vi "TestManager.vi"() -> ()   [LabVIEW 2018]
doc: "This is the central application/framework that controls module, run scripts, etc"
uses:
  TestConfigurationActions.ctl
  LV_Config_class/Config.lvclass/Config.ctl
  VisualizationManagement/VisualizationManagerActions.ctl
  NistPluggableModules/TestClass/Test.lvclass/Test.ctl
  <vilib>/Utility/miscctls.llb/LVRowAndColumnTypeDef.ctl
  LV_Config_class/Accessors/Read ConfigFilePath.vi
  LV_Config_class/Accessors/Write ConfigFilePath.vi
  NistPluggableModules/TestClass/Accessors/Read ModuleList.vi
  <vilib>/Utility/error.llb/Error Cluster From Error Code.vi
  <vilib>/ErrorRing/Error Ring.xnode
  Queue/Queue.lvlib
  <userlib>/NIST/NISTErrorLib/NISTErrorLib.lvlib
  LV_Config_class/Config.lvclass
  <vilib>/Utility/config.llb/NI_LVConfig.lvlib
  Message Queue/Message Queue.lvlib
  NistPluggableModules/TestClass/Test.lvclass
  LV_TestAutomation/Comms_lib/Comms.lvlib
panel:
  in  "Error In":errorcluster
  in  "Create Error (Test Python Multirun)":bool
  out "Test Tree Caption":string="Test Configuration"
  in  "btnClearTest":bool
  in  "btnSaveTestTree":bool
  in  "btnSaveTestAs":bool
  in  "btnLoadTest":bool
  in  "btnStopAllRunningTests":bool
  in  "btnRunAll":bool
  in  "TestTree":i32[](listbox)
  out "tstFilePath":path
  in  "Stop?":bool
  in  "btnRunScript":bool
  in  "btnDelete":bool
  out "OrigTestTreeTags":string[](array[string])
  out "Test Script":string
  in  "Experiment Specific Controls":T1(tab)
  in  "Priority":u8=2
  in  "Severity":string="Abort"
  out "Error Out":errorcluster
  in  "Severity":string
  in  "Priority":u8=2
  in  "Create Error (Test AutoTimeout)":bool
  in  "Error In 2":errorcluster
  # "Test Script Preview"
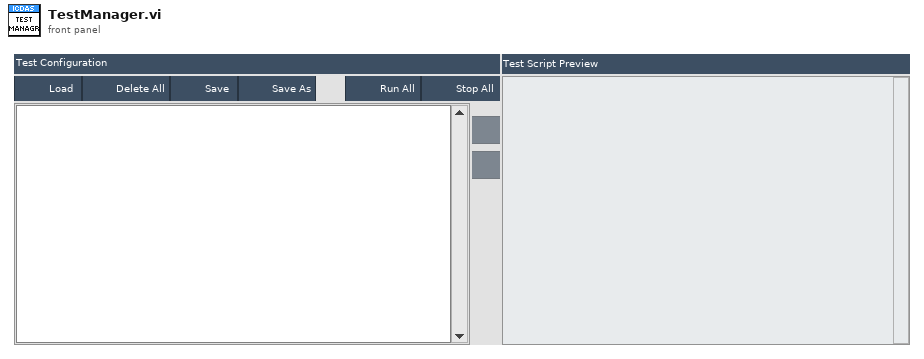
[diagram p1: front panel]
types:
  T1 = enum32{"PV Aging Experiment", "Pacific Power ", "Miscellaneous ", "Errors", "Test AutoTimeout", "Test Python MutliRun"}
  T2 = typedef "clUserEvents.ctl" = cluster{"StopEvent":refnum<user-event>, "RefreshUserEvents":refnum<user-event>, "StatusUpdate":refnum<user-event>, "RunAllScripts":refnum<user-event>}
  T3 = typedef "Message Queue.lvlib/All Message Queues.ctl" = cluster{"UI":refnum<queue>}
  T4 = typedef "cntlRefs.ctl" = cluster{"rngFGen":refnum<vi>, "rngDigitizer":refnum<vi>, "btnHide":refnum<vi>, "rngInst":refnum<vi>, "Instrument Modules":refnum<vi>, "RelativePathToINIFiles ":refnum<vi>, "PluginTree":refnum<vi>, "TestListboxRef":refnum<vi>, "path.tstFile":refnum<vi>, "cmbxRunningModules":refnum<vi>, "TestDataSubPanel":refnum<vi>, "TestDataCaption":refnum<vi>, "btnPopInOut":refnum<vi>, "PluginMgrQ":refnum<queue>, "TestMgrQ":refnum<queue>, "TestMgrSubPanel":refnum<vi>, "PluginMgrSubPanel":refnum<vi>, "PwrReqHandle":u32, "btnStopOneTest":refnum<vi>, "pathUserfiles":refnum<vi>, "PluginTreeCaption":refnum<vi>}
  T5 = enum8{"Enabled", "Disabled", "Disabled and Grayed Out"}
  T6 = typedef "TestConfigurationActions.ctl" = enum16{"Save", "Save As", "Read", "Read&Load"}
  T7 = typedef "VisualizationManagerActions.ctl" = enum16{"Set", "LoadModVI", "PopInOutModVI", "Add", "Clear", "CloseVisMod"}
  T8 = typedef "LVRowAndColumnTypeDef.ctl" = cluster{"Row":i32, "Column":i32}
  T9 = typedef "NI_LVConfig.lvlib/Config Data RefNum.ctl" = refnum<k1>
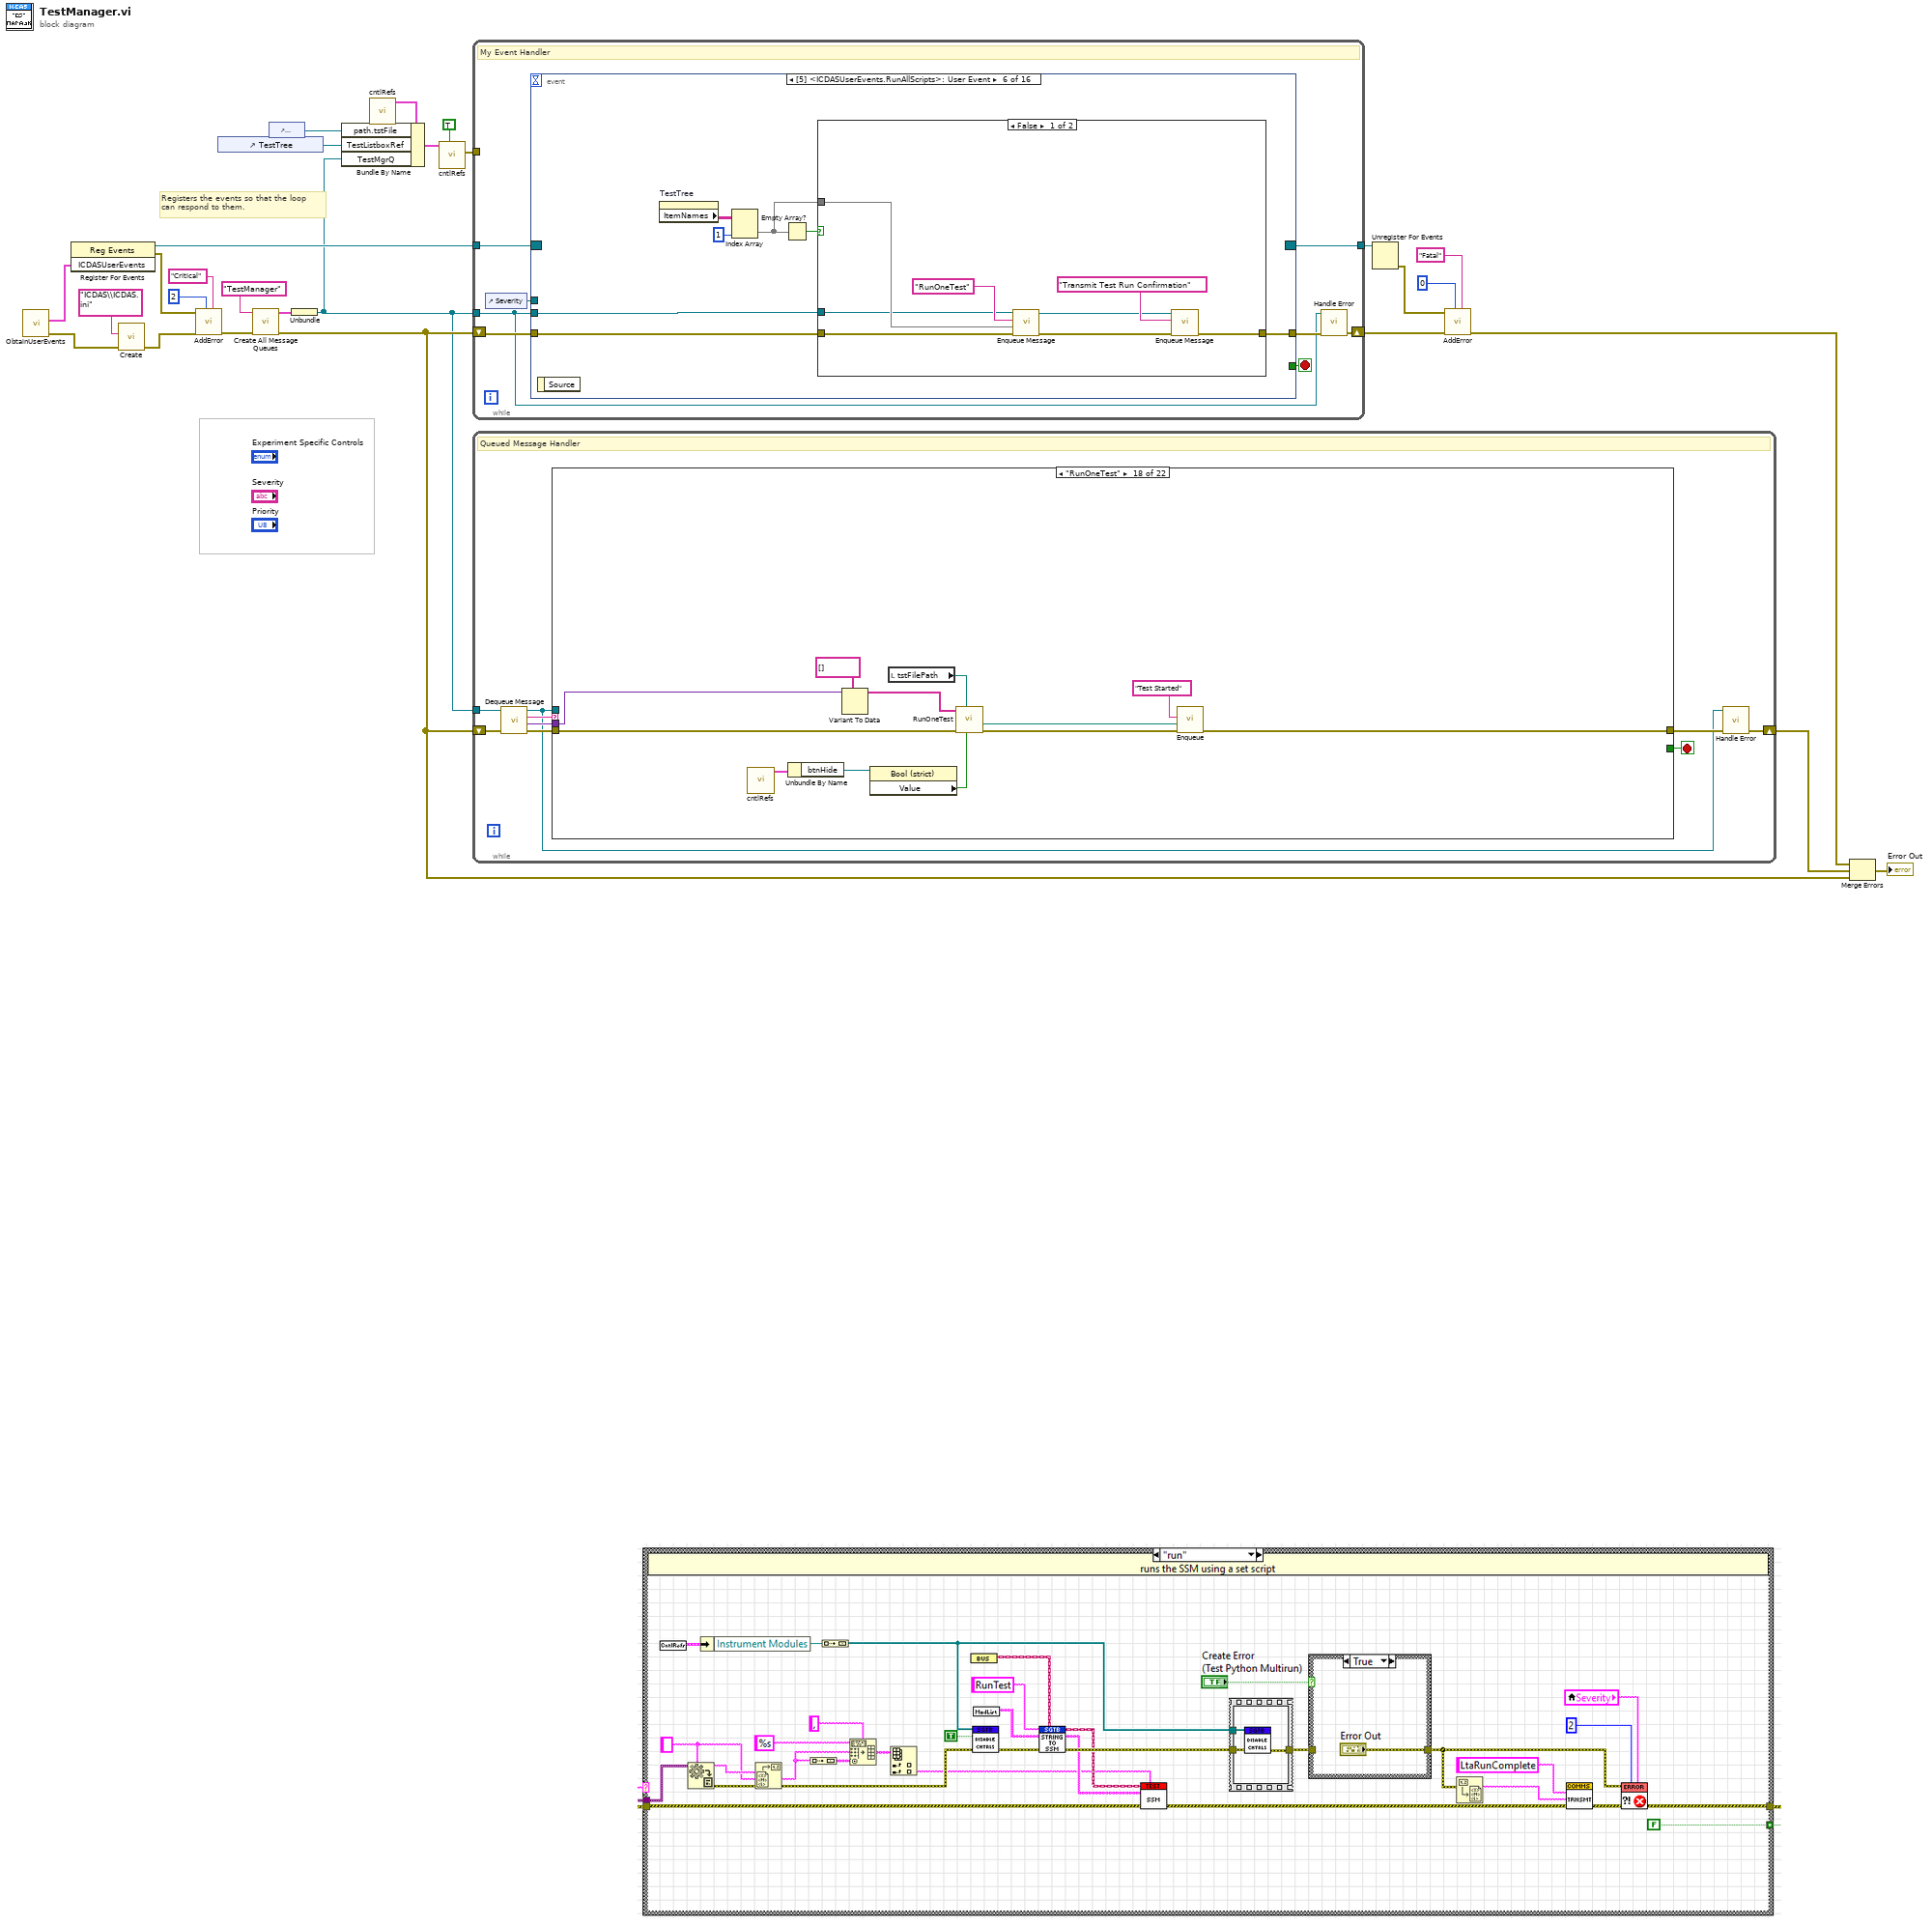
[diagram p0: block diagram]
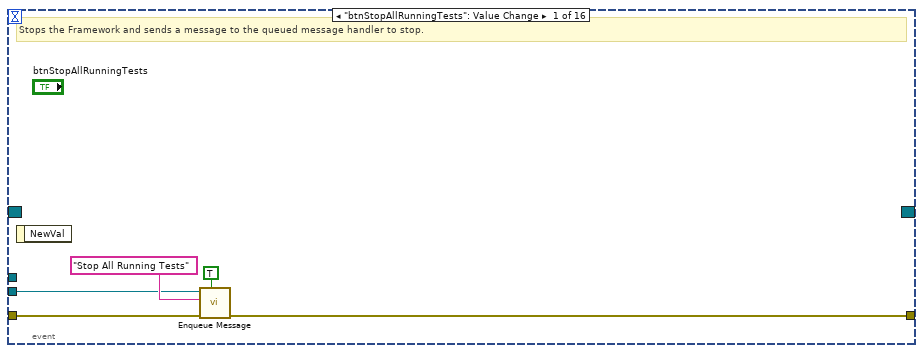
[diagram p2: hidden frame]
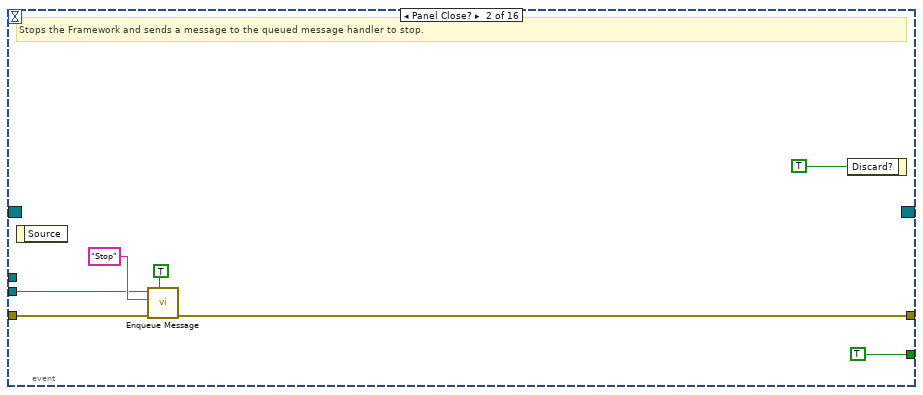
[diagram p3: hidden frame]
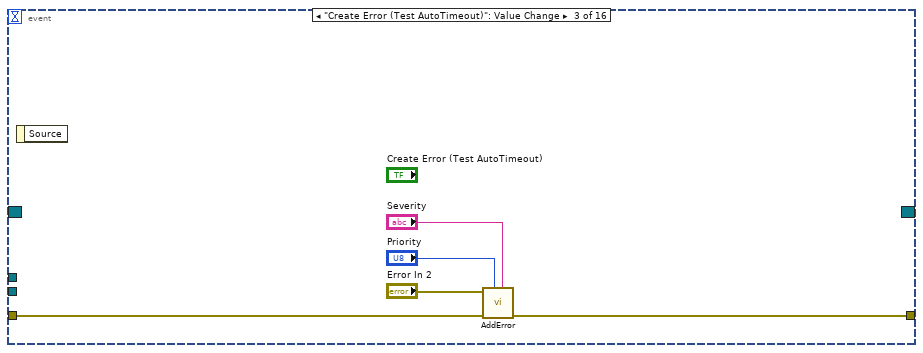
[diagram p4: hidden frame]
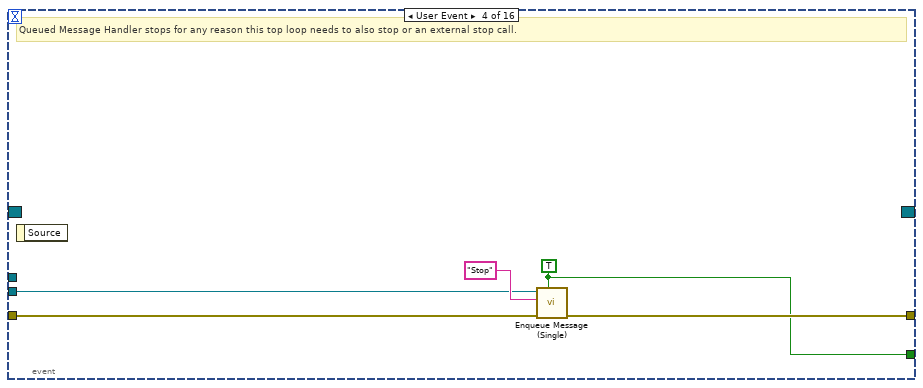
[diagram p5: hidden frame]
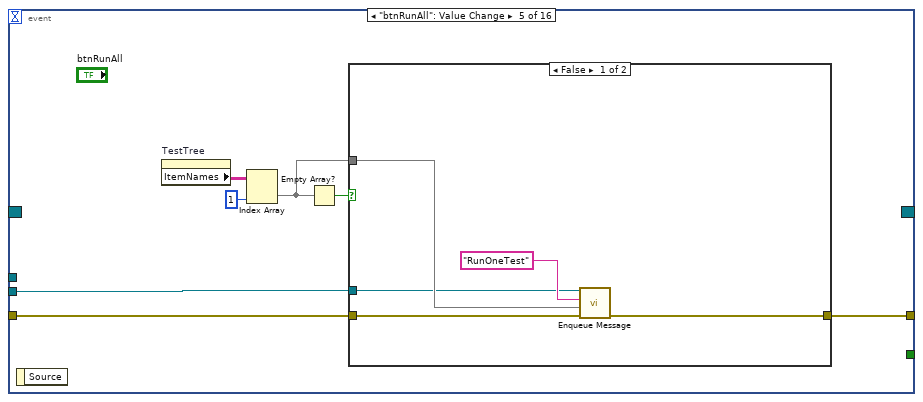
[diagram p6: hidden frame]
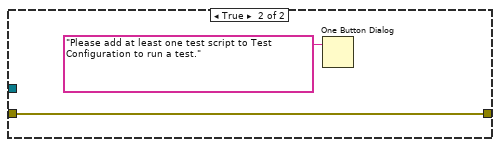
[diagram p7: hidden frame]
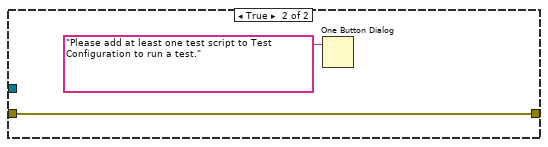
[diagram p8: hidden frame]
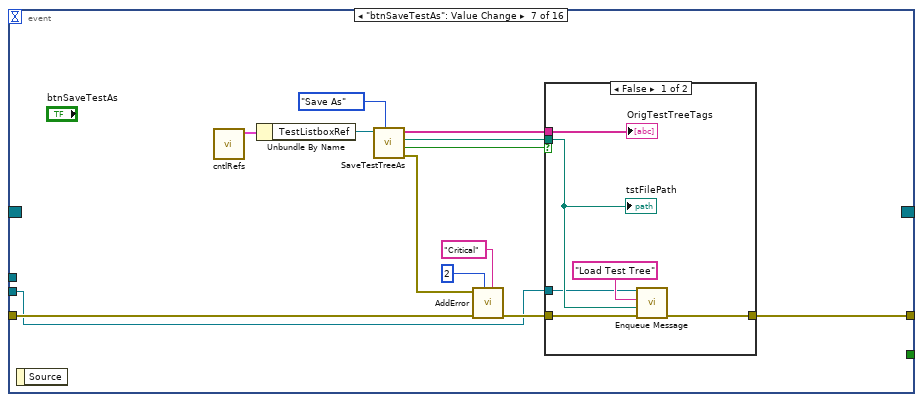
[diagram p9: hidden frame]
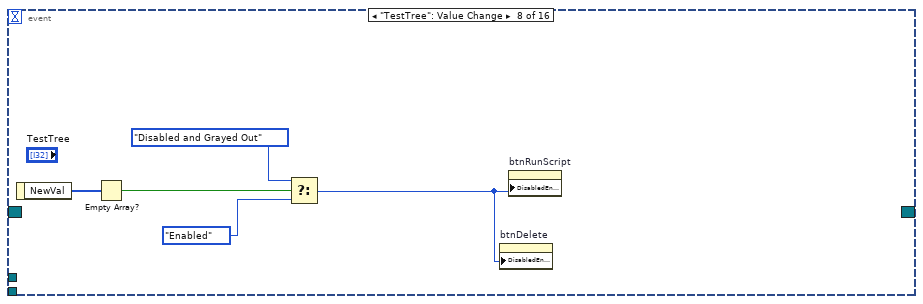
[diagram p11: hidden frame]
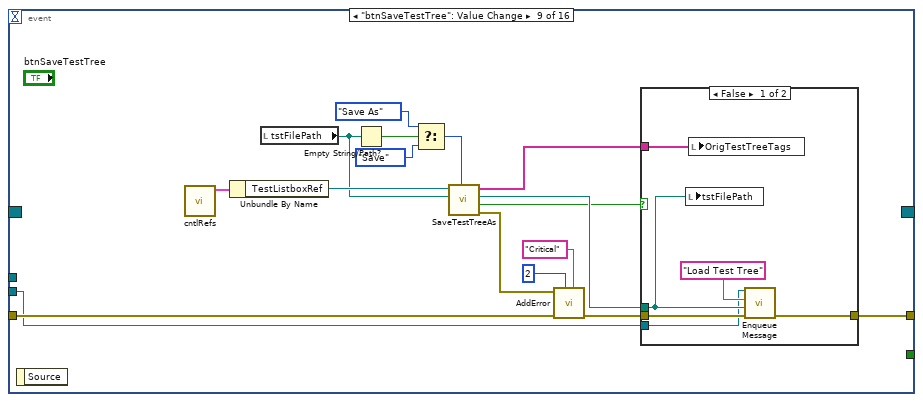
[diagram p12: hidden frame]
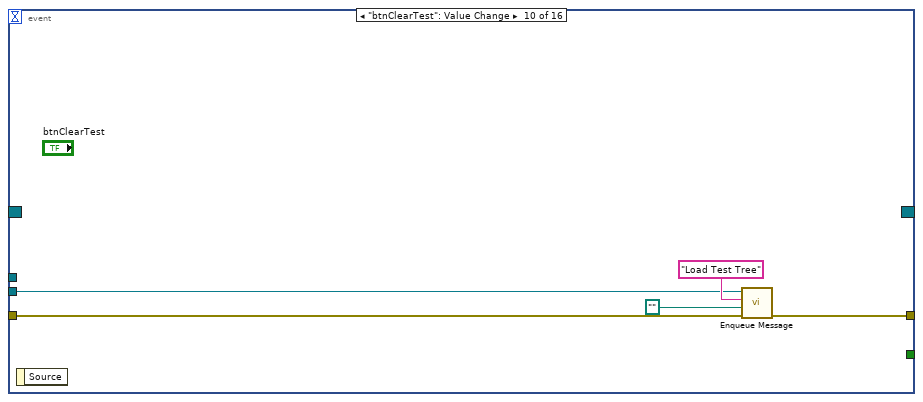
[diagram p14: hidden frame]
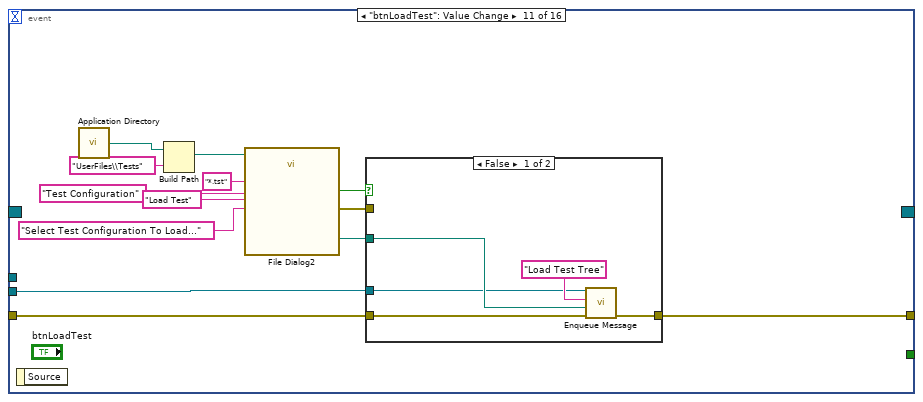
[diagram p15: hidden frame]
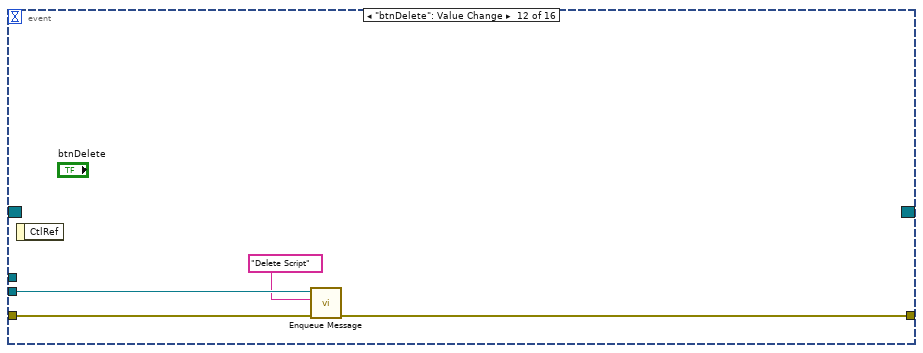
[diagram p17: hidden frame]
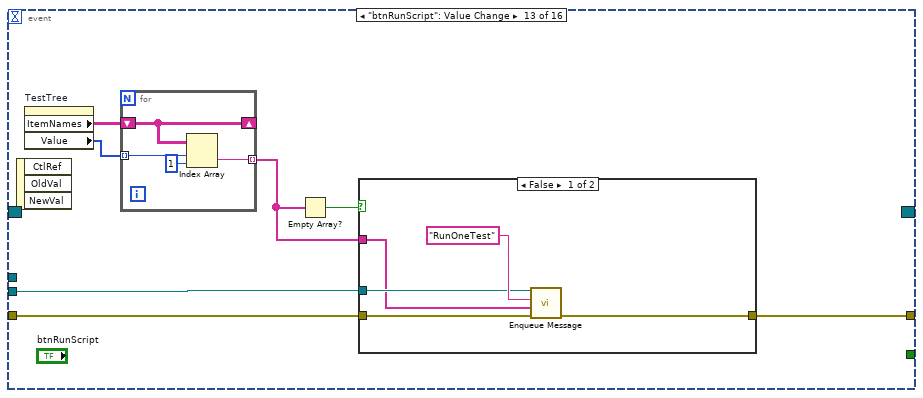
[diagram p18: hidden frame]
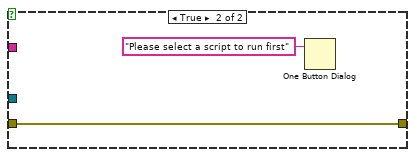
[diagram p19: hidden frame]
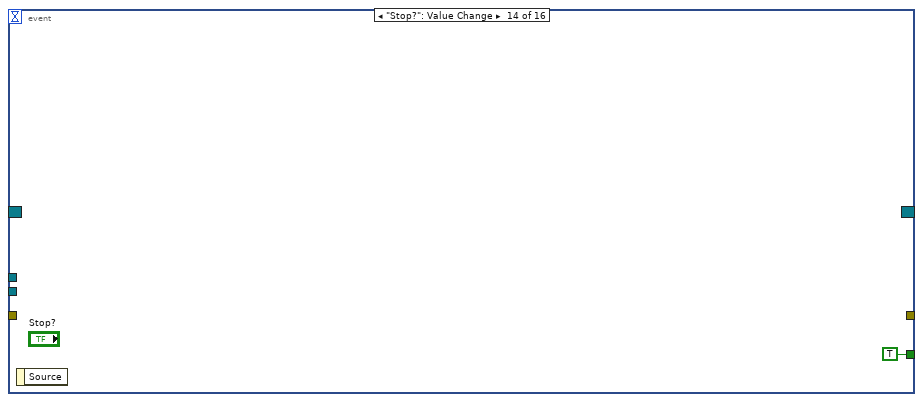
[diagram p20: hidden frame]
diagram:
  # "Registers the events so that the loop \ncan respond to them."
  n1 = call "ObtainUserEvents.vi"() -> ("ErrorArray"=w8:errorcluster[], "ICDASUserEvents"=w26:T2)  [unwired: 10 in]
  n2 = register-events(w26) -> (reference out=w27:refnum<event-registration>, error out=w16:errorcluster)  [unwired: 2 in]
  n3 = call "Create.vi"("ErrorArray"=w8, "name or relative path"="ICDAS\\ICDAS.ini") -> ("ErrorArray"=w7:errorcluster[])  [unwired: 8 in, 1 out]
  n4 = call <userlib>:"AddError.vi"("Severity"="Critical", "Priority"=u8 2, "ErrorArray In"=w7, "error in (no error)"=w16) -> ("ErrorArray Out"=w11:errorcluster[])  [unwired: 6 in, 1 out]
  n5 = control-ref of="TestTree"() -> (w15:refnum<vi>)
  n6 = call "Create All Message Queues.vi"("error in (no error)"=w11, "Queue Name (unnamed)"="TestManager") -> ("error out"=w10:errorcluster[], "Message Queues out"=w12:T3)  [unwired: 8 in]
  n7 = control-ref of="tstFilePath"() -> (w14:refnum<vi>)
  n8 = Unbundle(w12) -> ("UI"=w3:refnum<queue>)
  n9 = call "cntlRefs.vi"() -> ("cntlRefs"=w6:T4)  [unwired: 10 in, 1 out]
  n10 = Bundle By Name(cluster=w6, "path.tstFile"=w14, "TestListboxRef"=w15, "TestMgrQ"=w3) -> (w22:T4)
  n11 = call "cntlRefs.vi"("Set?"=TRUE, "cntlRefs"=w22) -> ("error out"=w4:errorcluster[])  [unwired: 8 in, 1 out]
  n12 = while {
    tunnel: w27 -> [w35]
    shift-right: [w33] -> w18
    shift-left: w10 -> [w34]
    tunnel: w3 -> [w29]
    tunnel: w4 -> [_]
    tunnel: [w28] -> w2
    stop <- w32 stop-if-true
    # "My Event Handler"
    n13 = control-ref of="Severity"() -> (w31:refnum<vi>)
    n14 = event shown="[5] <ICDASUserEvents.RunAllScripts>: User Event" {
      selector: w35 -> [_ _ _ _ _ _ _ _ _ _ _ _ _ _ _ _]
      dyn-events: [_ _ _ _ _ _ _ _ _ _ _ _ _ _ _ _] -> w28
      timeout: _ -> [_ _ _ _ _ _ _ _ _ _ _ _ _ _ _ _]
      tunnel: w34 -> [w40 w47 w51 w56 w63 w77 w96 _ w126 w142 w155 w164 w172 _ w188 w205]
      tunnel: [w37 w46 w50 w55 w62 w76 w93 _ w117 w141 w154 w165 w171 _ w187 w203] -> w30
      tunnel: [_ TRUE ("Priority (F)") _ w54 _ _ _ _ _ _ _ _ _ TRUE ("Priority (F)") _ _] -> w32
      tunnel: w31 -> [_ _ _ _ _ _ _ _ _ _ _ _ _ _ _ _]
      tunnel: w29 -> [w36 w41 _ w53 w61 w75 w89 _ w114 w138 w143 w163 w170 _ w186 w204]
      event "btnStopAllRunningTests": Value Change {
        # "Stops the Framework and sends a message to the queued message handler to stop."
        n15 = event-data() -> ()  [unwired: 1 in, 1 out]
        n16 = call-poly "Enqueue Message.vi"("Priority Message? (F)"=TRUE ("Priority (F)"), "error in (no error)"=w40, "Message"="Stop All Running Tests", "Message Queue"=w36) -> ("error out"=w37:errorcluster[])  [unwired: 6 in, 1 out]
      }
      event Panel Close? {
        # "Stops the Framework and sends a message to the queued message handler to stop."
        n17 = event-data() -> ()  [unwired: 1 in, 1 out]
        n18 = call-poly "Enqueue Message.vi"("Priority Message? (F)"=TRUE ("Priority (F)"), "error in (no error)"=w47, "Message"="Stop", "Message Queue"=w41) -> ("error out"=w46:errorcluster[])  [unwired: 6 in, 1 out]
        n19 = event-data("Discard?"=TRUE) -> ()  [unwired: 1 in, 1 out]
      }
      event "Create Error (Test AutoTimeout)": Value Change {
        n20 = event-data() -> ()  [unwired: 1 in, 1 out]
        n21 = call <userlib>:"AddError.vi"("Severity"="Severity", "Priority"="Priority", "ErrorArray In"=w51, "error in (no error)"="Error In 2") -> ("ErrorArray Out"=w50:errorcluster[])  [unwired: 6 in, 1 out]
      }
      event User Event {
        w54 = TRUE ("Priority (F)")
        # "Queued Message Handler stops for any reason this top loop needs to also stop or an external stop call."
        n22 = event-data() -> ()  [unwired: 1 in, 1 out]
        n23 = call "Enqueue Message (Single).vi"("Priority Message? (F)"=w54, "error in (no error)"=w56, "Message"="Stop", "Message Queue"=w53) -> ("error out"=w55:errorcluster[])  [unwired: 6 in, 1 out]
      }
      event "btnRunAll": Value Change {
        n24 = event-data() -> ()  [unwired: 1 in, 1 out]
        n25 = property on="TestTree" class="MCListbox (strict)"() -> ("ItemNames"=w60:string[][])  [unwired: 2 in, 2 out]
        n26 = Index Array(array=w60, index (col)=1 ("disabled index (col)")) -> (element=w58:string[])  [unwired: 1 in]
        n27 = Empty Array?(array=w58) -> (empty?=w64:bool)
        n28 = case shown="False" w64 {
          tunnel: w58 -> [w67 _]
          tunnel: w63 -> [w69 w70]
          tunnel: [w65 w70] -> w62
          tunnel: w61 -> [w66 _]
          frame False {
            n29 = call-poly "Enqueue Message.vi"("error in (no error)"=w69, "Message Data"=w67, "Message"="RunOneTest", "Message Queue"=w66) -> ("error out"=w65:errorcluster[])  [unwired: 6 in, 1 out]
          }
          frame True {
            n30 = One Button Dialog(message="Please add at least one test script to Test Configuration to run a test.") -> ()  [unwired: 1 in, 1 out]
          }
        }
      }
      event User Event {
        n31 = event-data() -> ()  [unwired: 1 in, 1 out]
        n32 = property on="TestTree" class="MCListbox (strict)"() -> ("ItemNames"=w74:string[][])  [unwired: 2 in, 2 out]
        n33 = Index Array(array=w74, index (col)=1 ("disabled index (col)")) -> (element=w72:string[])  [unwired: 1 in]
        n34 = Empty Array?(array=w72) -> (empty?=w78:bool)
        n35 = case shown="False" w78 {
          tunnel: w72 -> [w84 _]
          tunnel: w77 -> [w86 w87]
          tunnel: [w79 w87] -> w76
          tunnel: w75 -> [w83 _]
          frame False {
            n36 = call-poly "Enqueue Message.vi"("error in (no error)"=w86, "Message Data"=w84, "Message"="RunOneTest", "Message Queue"=w83) -> ("error out"=w80:errorcluster[], "dup Message Queue"=w81:refnum<queue>)  [unwired: 6 in]
            n37 = call-poly "Enqueue Message.vi"("error in (no error)"=w80, "Message"="Transmit Test Run Confirmation", "Message Queue"=w81) -> ("error out"=w79:errorcluster[])  [unwired: 7 in, 1 out]
          }
          frame True {
            n38 = One Button Dialog(message="Please add at least one test script to Test Configuration to run a test.") -> ()  [unwired: 1 in, 1 out]
          }
        }
      }
      event "btnSaveTestAs": Value Change {
        n39 = event-data() -> ()  [unwired: 1 in, 1 out]
        n40 = call "cntlRefs.vi"() -> ("cntlRefs"=w101:T4)  [unwired: 10 in, 1 out]
        n41 = Unbundle By Name(w101) -> ("TestListboxRef"=w100:refnum<vi>)
        n42 = call "SaveTestTreeAs.vi"("Action"=enum16{"Save", "Save As"}."Save As", "ListboxRef"=w100) -> ("error out"=w95:errorcluster, "Cancelled?"=w90:bool, "path.tstFile"=w92:path, "All Test Tree Tags"=w91:string[])  [unwired: 5 in, 1 out]
        n43 = call <userlib>:"AddError.vi"("Severity"="Critical", "Priority"=u8 2, "ErrorArray In"=w96, "error in (no error)"=w95) -> ("ErrorArray Out"=w94:errorcluster[])  [unwired: 6 in, 1 out]
        n44 = case shown="False" w90 {
          tunnel: w94 -> [w106 w108]
          tunnel: [w105 w108] -> w93
          tunnel: w92 -> [w104 _]
          tunnel: w91 -> [w103 _]
          tunnel: w89 -> [w102 _]
          frame False {
            n45 = call-poly "Enqueue Message.vi"("error in (no error)"=w106, "Message Data"=w104, "Message"="Load Test Tree", "Message Queue"=w102) -> ("error out"=w105:errorcluster[])  [unwired: 6 in, 1 out]
            "tstFilePath" <- w104
            "OrigTestTreeTags" <- w103
          }
          frame True {
          }
        }
      }
      event "TestTree": Value Change {
        n46 = event-data() -> ("NewVal"=w113:i32[])  [unwired: 1 in]
        n47 = Empty Array?(array=w113) -> (empty?=w112:bool)
        n48 = Select(t=T5."Disabled and Grayed Out" ("Disabled"), s=w112, f=T5."Enabled" ("Disabled")) -> (s? t:f=w109:T5)
        n49 = property on="btnDelete" class="Bool"("DisabledEnum"=w109) -> ()  [unwired: 2 in, 2 out]
        n50 = property on="btnRunScript" class="Bool"("DisabledEnum"=w109) -> ()  [unwired: 2 in, 2 out]
      }
      event "btnSaveTestTree": Value Change {
        n51 = event-data() -> ()  [unwired: 1 in, 1 out]
        n52 = call "cntlRefs.vi"() -> ("cntlRefs"=w129:T4)  [unwired: 10 in, 1 out]
        n53 = Unbundle By Name(w129) -> ("TestListboxRef"=w130:refnum<vi>)
        n54 = local read "tstFilePath"() -> (w124:path)
        n55 = Empty String/Path?(string/path=w124) -> (empty?=w123:bool)
        n56 = Select(t=TestConfigurationActions."Save As" ("Action"), s=w123, f=TestConfigurationActions."Save" ("Action")) -> (s? t:f=w120:T6)
        n57 = call "SaveTestTreeAs.vi"("Action"=w120, ".tst File Path"=w124, "ListboxRef"=w130) -> ("error out"=w125:errorcluster, "Cancelled?"=w115:bool, "path.tstFile"=w116:path, "All Test Tree Tags"=w119:string[])  [unwired: 4 in, 1 out]
        n58 = call <userlib>:"AddError.vi"("Severity"="Critical", "Priority"=u8 2, "ErrorArray In"=w126, "error in (no error)"=w125) -> ("ErrorArray Out"=w118:errorcluster[])  [unwired: 6 in, 1 out]
        n59 = case shown="False" w115 {
          tunnel: w119 -> [w136 _]
          tunnel: w118 -> [w134 w137]
          tunnel: [w133 w137] -> w117
          tunnel: w116 -> [w132 _]
          tunnel: w114 -> [w131 _]
          frame False {
            n60 = local write "tstFilePath"(w132) -> ()
            n61 = local write "OrigTestTreeTags"(w136) -> ()
            n62 = call-poly "Enqueue Message.vi"("error in (no error)"=w134, "Message Data"=w132, "Message"="Load Test Tree", "Message Queue"=w131) -> ("error out"=w133:errorcluster[])  [unwired: 6 in, 1 out]
          }
          frame True {
          }
        }
      }
      event "btnClearTest": Value Change {
        n63 = event-data() -> ()  [unwired: 1 in, 1 out]
        n64 = call-poly "Enqueue Message.vi"("error in (no error)"=w142, "Message Data"=path "", "Message"="Load Test Tree", "Message Queue"=w138) -> ("error out"=w141:errorcluster[])  [unwired: 6 in, 1 out]
      }
      event "btnLoadTest": Value Change {
        n65 = event-data() -> ()  [unwired: 1 in, 1 out]
        n66 = call <vilib>:"Application Directory.vi"() -> ("Application Directory"=w152:path)
        n67 = Build Path(base path=w152, name or relative path="UserFiles\\Tests") -> (appended path=w150:path)
        n68 = call "File Dialog2"("start path"=w150, "prompt"="Select Test Configuration To Load...", "button label"="Load Test", "pattern (all files)"="*.tst", "pattern label"="Test Configuration") -> ("selected path"=w145:path, "cancelled"=w144:bool, "error out"=w146:errorcluster)  [unwired: 7 in, 1 out]
        n69 = case shown="False" w144 {
          tunnel: w155 -> [w160 w161]
          tunnel: [w158 w161] -> w154
          tunnel: w146 -> [_ _]
          tunnel: w145 -> [w157 _]
          tunnel: w143 -> [w156 _]
          frame False {
            n70 = call-poly "Enqueue Message.vi"("error in (no error)"=w160, "Message Data"=w157, "Message"="Load Test Tree", "Message Queue"=w156) -> ("error out"=w158:errorcluster[])  [unwired: 6 in, 1 out]
          }
          frame True {
          }
        }
      }
      event "btnDelete": Value Change {
        n71 = event-data() -> ()  [unwired: 1 in, 1 out]
        n72 = call-poly "Enqueue Message.vi"("error in (no error)"=w164, "Message"="Delete Script", "Message Queue"=w163) -> ("error out"=w165:errorcluster[])  [unwired: 7 in, 1 out]
      }
      event "btnRunScript": Value Change {
        n73 = event-data() -> ()  [unwired: 1 in, 3 out]
        n74 = property on="TestTree" class="MCListbox (strict)"() -> ("ItemNames"=w169:string[][], "Value"=w168:i32[])  [unwired: 2 in, 2 out]
        n75 = for {
          shift-right: [w175] -> _
          shift-left: w169 -> [w175]
          tunnel: w168 -> [w176] mode=indexing
          tunnel: [w173] -> w167 mode=indexing
          n76 = Index Array(array=w175, index (row)=w176, index (col)=1 ("disabled index (col)")) -> (element=w173:string)
        }
        n77 = Empty Array?(array=w167) -> (empty?=w166:bool)
        n78 = case shown="False" w166 {
          tunnel: w172 -> [w181 w183]
          tunnel: [w180 w183] -> w171
          tunnel: w170 -> [w178 _]
          tunnel: w167 -> [w177 _]
          frame False {
            n79 = call-poly "Enqueue Message.vi"("error in (no error)"=w181, "Message Data"=w177, "Message"="RunOneTest", "Message Queue"=w178) -> ("error out"=w180:errorcluster[])  [unwired: 6 in, 1 out]
          }
          frame True {
            n80 = One Button Dialog(message="Please select a script to run first") -> ()  [unwired: 1 in, 1 out]
          }
        }
      }
      event "Stop?": Value Change {
        n81 = event-data() -> ()  [unwired: 1 in, 1 out]
      }
      event "TestTree": Drag Ended {
        n82 = event-data() -> ("Result"=w185:enum16{"Drop Cancel", "Drop Move", "Drop Copy"})  [unwired: 1 in]
        n83 = case shown="\"Drop Move\"" w185 {
          tunnel: w188 -> [w189 w195]
          tunnel: [w189 w194] -> w187
          tunnel: w186 -> [_ w193]
          frame "Drop Cancel", Default {
          }
          frame "Drop Move" {
            # "Refresh Test Script Preview"
            n84 = property on="TestTree" class="MCListbox (strict)"() -> ("ItemNames"=w192:string[][])  [unwired: 2 in, 2 out]
            n85 = Index Array(array=w192, index (col)=1 ("disabled index (col)")) -> (element=w190:string[])  [unwired: 1 in]
            n86 = local read "OrigTestTreeTags"() -> (w201:string[])
            n87 = call "CheckIfStringArraysAreEqual-1D.vi"("Array2"=w190, "Array1"=w201) -> ("Equal?"=w200:bool)  [unwired: 9 in]
            n88 = Not(x=w200) -> (.not. x?=w199:bool)
            n89 = call-poly "Enqueue Message.vi"("error in (no error)"=w195, "Message Data"=w199, "Message"="Test Tree Save State", "Message Queue"=w193) -> ("error out"=w202:errorcluster[], "dup Message Queue"=w198:refnum<queue>)  [unwired: 6 in]
            n90 = call-poly "Enqueue Message.vi"("error in (no error)"=w202, "Message"="Refresh Test Script", "Message Queue"=w198) -> ("error out"=w194:errorcluster[])  [unwired: 7 in, 1 out]
          }
        }
      }
      event Pane Size {
        n91 = event-data() -> ()  [unwired: 1 in, 6 out]
        n92 = call "Enqueue Message (Single).vi"("error in (no error)"=w205, "Message"="Resize Test Listbox Column", "Message Queue"=w204) -> ("error out"=w203:errorcluster[])  [unwired: 7 in, 1 out]
      }
    }
    n93 = call "Handle Error.vi"("ErrorArrayIn"=w30, "Message Queue"=w29) -> ("ErrorArrayOut"=w33:errorcluster[])  [unwired: 9 in]
  }
  n94 = while {
    shift-right: [w214] -> w21
    shift-left: w10 -> [w209]
    tunnel: w3 -> [w212]
    stop <- w213 stop-if-true
    # "Queued Message Handler"
    n95 = call "Dequeue Message.vi"("error in (no error)"=w209, "Message Queue"=w212) -> ("error out"=w208:errorcluster[], "Message Data"=w211:variant, "Message"=w210:string, "dup Message Queue"=w207:refnum<queue>)  [unwired: 6 in]
    n96 = case shown="\"RunOneTest\"" w210 {
      selector: w210 -> [_ _ _ _ _ _ w377 _ _ _ _ _ _ _ _ _ _ _ _ _ _ _]
      tunnel: [w229 w266 w269 w311 w356 w368 w376 w385 w394 w398 w411 w472 w476 w481 w503 w505 w548 w550 w562 w569 w576 w583] -> w215
      tunnel: w208 -> [w236 w265 w274 w310 w351 w359 w375 w385 w394 w397 w431 w471 w476 w482 w503 w515 w548 w556 w564 w568 w576 w583]
      tunnel: [_ _ _ _ _ TRUE _ _ _ _ _ _ _ _ _ _ _ _ _ _ _ _] -> w213
      tunnel: w211 -> [_ w264 w275 _ w355 _ _ _ w392 _ w425 _ _ w478 _ w514 _ w557 _ _ _ _]
      tunnel: w207 -> [w225 w263 w267 w301 w333 w364 _ _ _ _ w407 w470 _ w480 _ _ _ _ _ _ _ _]
      frame "Initialize" {
        # "Pulls the default configuration from the INI file"
        n97 = call "GetSetConfigClass.vi"() -> ("Ref out"=w234:refnum<class "Config.lvclass">)  [unwired: 11 in]
        n98 = property class="Config.lvclass"(reference=w234) -> ("Accessors:ConfigFilePath"=w231:path)  [unwired: 1 in, 2 out]
        n99 = To Variant(anything=w231) -> (Variant=w230:variant)
        n100 = call "cntlRefs.vi"() -> ("cntlRefs"=w228:T4)  [unwired: 10 in, 1 out]
        n101 = Unbundle By Name(w228) -> ("TestListboxRef"=w224:refnum<vi>)
        n102 = call "Enqueue Message (Single).vi"("error in (no error)"=w236, "Message Data"=w230, "Message"="LoadTest", "Message Queue"=w225) -> ("error out"=w219:errorcluster[], "dup Message Queue"=w217:refnum<queue>)  [unwired: 6 in]
        n103 = call "Enqueue Message (Single).vi"("error in (no error)"=w219, "Message"="Resize Test Listbox Column", "Message Queue"=w217) -> ("error out"=w218:errorcluster[])  [unwired: 7 in, 1 out]
        n104 = property class="MCListbox"(reference=w224, "ItemNames"=string[][] [] ("Item Names")) -> (reference out=w223:refnum<vi>, error out=w221:errorcluster)  [unwired: 1 in]
        n105 = call "ListboxSymbols-FG.vi"("Actions"=enum16{"Init Symbols", "Set Item Symbol"}."Init Symbols", "error in (no error)"=w221, "ListboxRef"=w223) -> ("error out"=w220:errorcluster)  [unwired: 5 in, 3 out]
        n106 = call <userlib>:"AddError.vi"("Severity"="Fatal", "Priority"=u8 0, "ErrorArray In"=w218, "error in (no error)"=w220) -> ("ErrorArray Out"=w229:errorcluster[])  [unwired: 6 in, 1 out]
        "Test Script" <- ""
      }
      frame "LoadTest" {
        # "From the default file load the last saved results and updated the controls and indicators"
        n107 = call "cntlRefs.vi"() -> ("cntlRefs"=w258:T4)  [unwired: 10 in, 1 out]
        n108 = Variant To Data(type=path "", Variant=w264) -> (data=w260:path, error out=w262:errorcluster)  [unwired: 1 in]
        n109 = Unbundle By Name(w258) -> ("path.tstFile"=w257:refnum<vi>)
        n110 = call <vilib>:"Open Config Data.vi"("error in (no error)"=w262, "configuration file path"=w260) -> ("error out"=w241:errorcluster, "refnum"=w259:T9)  [unwired: 7 in, 1 out]
        n111 = property class="Path"(reference=w257, error in=w241) -> (error out=w254:errorcluster, "Label.Text"=w255:string)  [unwired: 1 out]
        n112 = call <userlib>:"Read Key (Variant)__ogtk.vi"("section"=w255, "error in (no error)"=w254, "type"=w255, "key (optional)"=w255, "refnum"=w259) -> ("error out"=w253:errorcluster, "key-value"=w256:variant, "refnum out"=w240:T9)  [unwired: 3 in, 1 out]
        n113 = Variant To Data(error in=w253, type=w255, Variant=w256) -> (data=w252:string, error out=w239:errorcluster)
        n114 = call <vilib>:"Trim Whitespace.vi"("string"=w252) -> ("trimmed string"=w246:string)  [unwired: 1 in]
        n115 = call <vilib>:"Close Config Data.vi"("error in (no error)"=w239, "write file if changed (T)"=FALSE, "refnum"=w240) -> ("error out"=w238:errorcluster)  [unwired: 7 in, 1 out]
        n116 = Empty String/Path?(string/path=w246) -> (empty?=w245:bool)
        n117 = call <vilib>:"Application Directory.vi"() -> ("Application Directory"=w247:path)
        n118 = local read "Severity"() -> (w250:string)
        n119 = local read "Priority"() -> (w251:u8)
        n120 = Build Path(base path=w247, name or relative path=w246) -> (appended path=w243:path)
        n121 = Select(t=path "", s=w245, f=w243) -> (s? t:f=w242:path)
        n122 = call <userlib>:"AddError.vi"("Severity"=w250, "Priority"=w251, "ErrorArray In"=w265, "error in (no error)"=w238) -> ("ErrorArray Out"=w249:errorcluster[])  [unwired: 6 in, 1 out]
        n123 = call-poly "Enqueue Message.vi"("error in (no error)"=w249, "Message Data"=w242, "Message"="Load Test Tree", "Message Queue"=w263) -> ("error out"=w266:errorcluster[])  [unwired: 6 in, 1 out]
      }
      frame "Error" {
        n124 = Variant To Data(type=w274, Variant=w275) -> (data=w273:errorcluster[], error out=w268:errorcluster)  [unwired: 1 in]
        n125 = call <userlib>:"ParseErrors.vi"("ErrorArray"=w273) -> ("ErrorArray"=w276:errorcluster[])  [unwired: 8 in, 2 out]
        n126 = for {
          tunnel: w276 -> [w283] mode=indexing
          tunnel: [w286] -> w270 mode=concatenating
          tunnel: w267 -> [w277]
          n127 = call <userlib>:"GeneralHandler.vi"("error in (no error)"=w283) -> ("Severity"=w284:string, "Stop"=w280:bool, "Abort"=w281:bool, "Continue"=w282:bool, "Error Out"=w278:errorcluster)  [unwired: 6 in]
          n128 = Build Array(w282, w281, w280) -> (w279:bool[])
          n129 = Boolean Array To Number(Boolean array=w279) -> (number=w285:u32)
          n130 = case shown="2" w285 {
            tunnel: w284 -> [_ _ _ _]
            tunnel: [_ _ w288 w300] -> w286
            tunnel: w283 -> [_ _ _ _]
            tunnel: w278 -> [_ _ w290 _]
            tunnel: w277 -> [_ _ w287 _]
            frame 0, Default {
              # "No Dialog"
            }
            frame 1 {
              # "Continue"
            }
            frame 2 {
              # "Abort Button Pressed"
              n131 = Flush Queue(queue=w287, error in (no error)=w290) -> (error out=w293:errorcluster)  [unwired: 2 out]
              n132 = call <userlib>:"AddError.vi"("Severity"="Critical", "Priority"=u8 1, "error in (no error)"=w293) -> ("ErrorArray Out"=w289:errorcluster[])  [unwired: 7 in, 1 out]
              n133 = disable-structure shown="Disabled" {
                disable-tunnel: w289 -> [w296 w299]
                disable-tunnel: [w295 w299] -> w288
                frame Disabled {
                  n134 = To Variant(anything="*AbortScript" ("Message")) -> (Variant=w297:variant)
                  n135 = call "Enqueue.vi"("ErrorArray"=w296, "Message Data"=w297, "Message"="RunOneTest") -> ("ErrorArray"=w295:errorcluster[])  [unwired: 8 in]
                }
                frame Enabled {
                }
              }
            }
            frame 4 {
              # "Stop this application"
              n136 = call "StopEvent.vi"() -> ("ErrorArray"=w300:errorcluster[])  [unwired: 11 in]
            }
          }
        }
        n137 = call <userlib>:"AddError.vi"("Severity"="Fatal", "Priority"=u8 0, "ErrorArray In"=w270, "error in (no error)"=w268) -> ("ErrorArray Out"=w269:errorcluster[])  [unwired: 6 in, 1 out]
      }
      frame "Stop" {
        n138 = disable-structure shown="Enabled" {
          disable-tunnel: [w330 FALSE ("T button?")] -> w306
          frame Disabled {
            n139 = Two Button Dialog(message="Save Application configuration to a new location?") -> (T button?=w330:bool)  [unwired: 2 in]
          }
          frame Enabled {
          }
        }
        n140 = call "GetSetConfigClass.vi"() -> ("Ref out"=w314:refnum<class "Config.lvclass">)  [unwired: 11 in]
        n141 = property class="Config.lvclass"(reference=w314) -> (reference out=w304:refnum<class "Config.lvclass">, error out=w307:errorcluster, "Accessors:ConfigFilePath"=w308:path)  [unwired: 1 in]
        n142 = case shown="True" w306 {
          tunnel: w308 -> [w315 w326]
          tunnel: w307 -> [w316 w325]
          tunnel: [w316 w317] -> w305
          tunnel: w304 -> [_ w321]
          tunnel: [w315 w318] -> w303
          frame False {
          }
          frame True {
            n143 = call "FileDialog.vi"("Error In"=w325, "File Path Control In"=w326) -> ("Error Out"=w323:errorcluster, "Valid File Path?"=w320:bool, "File Path Control Out"=w319:path)  [unwired: 7 in]
            n144 = Select(t=w319, s=w320, f=w326) -> (s? t:f=w324:path)
            n145 = property class="Config.lvclass"(reference=w321, error in=w323, "Accessors:ConfigFilePath"=w324) -> (reference out=w322:refnum<class "Config.lvclass">, error out=w317:errorcluster, "Accessors:ConfigFilePath"=w318:path)
            n146 = flat-sequence {
              tunnel: w322 -> [w329]
              tunnel: w317 -> [_]
              frame #0 {
                n147 = Two Button Dialog(message="Update configuration file path") -> (T button?=w328:bool)  [unwired: 2 in]
                n148 = call "GetSetConfigClass.vi"("Set (f)"=w328, "Ref in"=w329) -> ()  [unwired: 9 in, 1 out]
              }
            }
          }
        }
        n149 = local read "Severity"() -> (w302:string)
        n150 = call "Enqueue Message (Single).vi"("error in (no error)"=w310, "Message Data"=w303, "Message"="SaveTest", "Message Queue"=w301) -> ("error out"=w309:errorcluster[])  [unwired: 6 in, 1 out]
        n151 = call <userlib>:"AddError.vi"("Severity"=w302, "Priority"=u8 0, "ErrorArray In"=w309, "error in (no error)"=w305) -> ("ErrorArray Out"=w311:errorcluster[])  [unwired: 6 in, 1 out]
      }
      frame "SaveTest" {
        # "saves the state of the controls and indicators into an INI file"
        n152 = Variant To Data(type=path "", Variant=w355) -> (data=w350:path, error out=w354:errorcluster)  [unwired: 1 in]
        n153 = call "cntlRefs.vi"() -> ("cntlRefs"=w347:T4)  [unwired: 10 in, 1 out]
        n154 = call <vilib>:"Open Config Data.vi"("error in (no error)"=w354, "configuration file path"=w350) -> ("error out"=w353:errorcluster, "refnum"=w349:T9)  [unwired: 7 in, 1 out]
        n155 = Unbundle By Name(w347) -> ("path.tstFile"=w343:refnum<vi>)
        n156 = call <userlib>:"AddError.vi"("ErrorArray In"=w351, "error in (no error)"=w353) -> ("ErrorArray Out"=w352:errorcluster[])  [unwired: 8 in, 1 out]
        n157 = property class="Path"(reference=w343) -> (error out=w339:errorcluster, "Label.Text"=w340:string, "Value"=w338:path)  [unwired: 1 in, 1 out]
        n158 = call "ConvertAbsolutePathToRelative.vi"("Absolute Path"=w338) -> ("RelativePath"=w337:string)  [unwired: 10 in]
        n159 = call <userlib>:"Write Key (Variant)__ogtk.vi"("section"=w340, "error in (no error)"=w339, "key-value"=w337, "key (optional)"=w340, "refnum"=w349) -> ("error out"=w335:errorcluster, "refnum out"=w336:T9)  [unwired: 5 in]
        n160 = call <vilib>:"Close Config Data.vi"("error in (no error)"=w335, "write file if changed (T)"=TRUE, "refnum"=w336) -> ("error out"=w334:errorcluster)  [unwired: 7 in, 1 out]
        n161 = call <userlib>:"AddError.vi"("Severity"="Abort", "Priority"=u8 3, "ErrorArray In"=w352, "error in (no error)"=w334) -> ("ErrorArray Out"=w345:errorcluster[])  [unwired: 6 in, 1 out]
        n162 = call-poly "Enqueue Message.vi"("error in (no error)"=w345, "Message"="End", "Message Queue"=w333) -> ("error out"=w356:errorcluster[])  [unwired: 7 in, 1 out]
      }
      frame "End" {
        n163 = Release Queue(queue=w364, force destroy? (F)=TRUE) -> (error out=w363:errorcluster)  [unwired: 1 in, 2 out]
        n164 = call "GetSetTestClass.vi"() -> ("Test.lvclass"=w361:refnum<class "Test.lvclass">)  [unwired: 11 in]
        n165 = call "StopMods.vi"("ErrorArray In"=w359, "Test.lvclass"=w361) -> ("ErrorArray Out"=w360:errorcluster[])  [unwired: 8 in, 1 out]
        n166 = property on="Stop?" class="Bool (strict)"("Val(Sgnl)"=TRUE ("Value (Signaling)")) -> ()  [unwired: 2 in, 2 out]
        n167 = call <userlib>:"AddError.vi"("Severity"="Abort", "Priority"=u8 3, "ErrorArray In"=w360, "error in (no error)"=w363) -> ("ErrorArray Out"=w368:errorcluster[])  [unwired: 6 in, 1 out]
        n168 = call "cntlRefs.vi"() -> ("cntlRefs"=w367:T4)  [unwired: 10 in, 1 out]
        n169 = Unbundle By Name(w367) -> ("TestListboxRef"=w366:refnum<vi>)
        n170 = local write "Test Script"("") -> ()
        n171 = property class="MCListbox"(reference=w366, "ItemNames"=string[][] [] ("Item Names")) -> ()  [unwired: 1 in, 2 out]
      }
      frame Default {
        n172 = xnode "Error Ring"("parameter 0"=w377) -> ("error out"=w372:errorcluster)
        n173 = call <userlib>:"AddError.vi"("Severity"="Inform", "Priority"=u8 5, "ErrorArray In"=w375, "error in (no error)"=w372) -> ("ErrorArray Out"=w376:errorcluster[])  [unwired: 6 in, 1 out]
      }
      frame "----Test Setup----" {
      }
      frame "Test Tree Save State" {
        w387 = "*" ("string")
        n174 = Variant To Data(type=FALSE, Variant=w392) -> (data=w390:bool)  [unwired: 1 in, 1 out]
        n175 = local read "Test Tree Caption"() -> (w388:string)
        n176 = Match Pattern(string=w388, regular expression=w387) -> (before substring=w386:string)  [unwired: 1 in, 3 out]
        n177 = Concatenate Strings(w386, w387) -> (w391:string)
        n178 = Select(t=w391, s=w390, f=w386) -> (s? t:f=w389:string)
        n179 = local write "Test Tree Caption"(w389) -> ()
      }
      frame "Refresh Test Script" {
        n180 = call "cntlRefs.vi"() -> ("cntlRefs"=w403:T4)  [unwired: 10 in, 1 out]
        n181 = Unbundle By Name(w403) -> ("TestListboxRef"=w402:refnum<vi>)
        n182 = call "RefreshTestTreeScript.vi"("TestListboxRef"=w402) -> ("error out"=w396:errorcluster, "String"=w401:string)  [unwired: 9 in]
        n183 = property on="Test Script" class="Str"(error in=w396, "Value"=w401) -> (error out=w395:errorcluster)  [unwired: 1 in, 1 out]
        n184 = call <userlib>:"AddError.vi"("Severity"="Critical", "Priority"=u8 2, "ErrorArray In"=w397, "error in (no error)"=w395) -> ("ErrorArray Out"=w398:errorcluster[])  [unwired: 6 in, 1 out]
      }
      frame "Load Test Tree" {
        w418 = "Test Configuration" ("format string")
        # "Trigger delete button enable/disable"
        n185 = call "cntlRefs.vi"() -> ("cntlRefs"=w415:T4)  [unwired: 10 in, 1 out]
        n186 = Unbundle By Name(w415) -> ("TestListboxRef"=w414:refnum<vi>)
        n187 = Variant To Data(type=path "", Variant=w425) -> (data=w422:path, error out=w423:errorcluster)  [unwired: 1 in]
        n188 = Empty String/Path?(string/path=w422) -> (empty?=w421:bool)
        n189 = case shown="False" w421 {
          tunnel: [w438 w442] -> w428
          tunnel: [w436 _] -> w409
          tunnel: w422 -> [w435 _]
          tunnel: w423 -> [w434 w441]
          tunnel: w414 -> [w432 w443]
          tunnel: [w433 _] -> w408
          tunnel: [w432 w440] -> _
          frame False {
            n190 = call "SaveTestTreeAs.vi"("Action"=TestConfigurationActions."Read&Load", "error in (no error)"=w434, ".tst File Path"=w435, "ListboxRef"=w432) -> ("error out"=w438:errorcluster, "path.tstFile"=w436:path, "All Test Tree Tags"=w433:string[])  [unwired: 3 in, 2 out]
          }
          frame True {
            # "Clear tree"
            n191 = property class="MCListbox"(reference=w443, error in=w441, "ItemNames"=string[][] [] ("Item Names")) -> (reference out=w440:refnum<vi>, error out=w442:errorcluster)
          }
        }
        n192 = local write "OrigTestTreeTags"(w408) -> ()
        n193 = call <userlib>:"AddError.vi"("Severity"="Critical", "Priority"=u8 2, "ErrorArray In"=w431, "error in (no error)"=w428) -> ("ErrorArray Out"=w426:errorcluster[])  [unwired: 6 in, 1 out]
        n194 = local write "tstFilePath"(w409) -> ()
        n195 = Strip Path(path=w409) -> (name=w419:string)  [unwired: 1 out]
        n196 = call-poly "Enqueue Message.vi"("error in (no error)"=w426, "Message"="Refresh Test Script", "Message Queue"=w407) -> ("error out"=w412:errorcluster[], "dup Message Queue"=w406:refnum<queue>)  [unwired: 7 in]
        n197 = Empty String/Path?(string/path=w409) -> (empty?=w416:bool)
        n198 = Concatenate Strings(w418, " - " ("string"), w419) -> (w417:string)
        n199 = Select(t=w418, s=w416, f=w417) -> (s? t:f=→"Test Tree Caption":string)
        n200 = call-poly "Enqueue Message.vi"("error in (no error)"=w412, "Message Data"=FALSE, "Message"="Test Tree Save State", "Message Queue"=w406) -> ("error out"=w411:errorcluster[])  [unwired: 6 in, 1 out]
        n201 = property on="TestTree" class="MCListbox (strict)"() -> ("Value"=w404:i32[])  [unwired: 2 in, 2 out]
        n202 = property on="TestTree" class="MCListbox (strict)"("Val(Sgnl)"=w404) -> ()  [unwired: 2 in, 2 out]
      }
      frame "Delete Script" {
        n203 = call "cntlRefs.vi"() -> ("cntlRefs"=w469:T4)  [unwired: 10 in, 1 out]
        n204 = Unbundle By Name(w469) -> ("TestListboxRef"=w459:refnum<vi>)
        n205 = property on="TestTree" class="MCListbox (strict)"() -> ("Value"=w454:i32[])  [unwired: 2 in, 2 out]
        n206 = property class="MCListbox"(reference=w459) -> (reference out=w461:refnum<vi>, error out=w460:errorcluster, "ItemNames"=w452:string[][], "ItemSyms"=w447:i32[])  [unwired: 1 in]
        n207 = Sort 1D Array(array=w454) -> (sorted array=w453:i32[])
        n208 = Reverse 1D Array(array=w453) -> (reversed array=w451:i32[])
        n209 = for {
          shift-right: [w473] -> w449
          shift-left: w452 -> [w475]
          tunnel: w451 -> [w474] mode=indexing
          n210 = Delete From Array(array=w475, index (row)=w474) -> (array with subset deleted=w473:string[][])  [unwired: 2 in, 1 out]
        }
        n211 = Index Array(array=w449, index (col)=1 ("disabled index (col)")) -> (element=w448:string[])  [unwired: 1 in]
        n212 = Array Size(array=w448) -> (size(s)=w446:i32)
        n213 = Array Subset(array=w447, index=0, length=w446) -> (w444:i32[])
        n214 = property class="MCListbox"(reference=w461, error in=w460, "ItemNames"=w449, "ItemSyms"=w444) -> (error out=w462:errorcluster)  [unwired: 1 out]
        n215 = local read "OrigTestTreeTags"() -> (w468:string[])
        n216 = call <userlib>:"AddError.vi"("Severity"="Critical", "Priority"=u8 2, "ErrorArray In"=w471, "error in (no error)"=w462) -> ("ErrorArray Out"=w457:errorcluster[])  [unwired: 6 in, 1 out]
        n217 = call "CheckIfStringArraysAreEqual-1D.vi"("Array2"=w448, "Array1"=w468) -> ("Equal?"=w466:bool)  [unwired: 9 in]
        n218 = call-poly "Enqueue Message.vi"("error in (no error)"=w457, "Message"="Refresh Test Script", "Message Queue"=w470) -> ("error out"=w456:errorcluster[], "dup Message Queue"=w455:refnum<queue>)  [unwired: 7 in]
        n219 = Not(x=w466) -> (.not. x?=w465:bool)
        n220 = call-poly "Enqueue Message.vi"("error in (no error)"=w456, "Message Data"=w465, "Message"="Test Tree Save State", "Message Queue"=w455) -> ("error out"=w472:errorcluster[])  [unwired: 6 in, 1 out]
      }
      frame "----Messages From Plugin Manager----" {
      }
      frame "Add Script to Test" {
        n221 = call "cntlRefs.vi"() -> ("cntlRefs"=w483:T4)  [unwired: 10 in, 1 out]
        n222 = Variant To Data(type="", Variant=w478) -> (data=w477:string)  [unwired: 1 in, 1 out]
        n223 = Unbundle By Name(w483) -> ("TestListboxRef"=w487:refnum<vi>)
        n224 = call "CopyScriptFromPluginTreeToTestTree.vi"("Script Tag to Add to Test"=w477, "TestListboxRef"=w487) -> ("error out"=w486:errorcluster, "Added Script?"=w489:bool, "All Tags"=w490:string[])  [unwired: 7 in]
        n225 = call <userlib>:"AddError.vi"("Severity"="Critical", "Priority"=u8 2, "ErrorArray In"=w482, "error in (no error)"=w486) -> ("ErrorArray Out"=w488:errorcluster[])  [unwired: 6 in, 1 out]
        n226 = case shown="True" w489 {
          tunnel: w488 -> [w491 w499]
          tunnel: [w491 w501] -> w481
          tunnel: w490 -> [_ w495]
          tunnel: w480 -> [_ w493]
          frame False {
          }
          frame True {
            # "Refresh Test Script Preview"
            n227 = local read "OrigTestTreeTags"() -> (w497:string[])
            n228 = call "CheckIfStringArraysAreEqual-1D.vi"("Array2"=w495, "Array1"=w497) -> ("Equal?"=w496:bool)  [unwired: 9 in]
            n229 = Not(x=w496) -> (.not. x?=w494:bool)
            n230 = call-poly "Enqueue Message.vi"("error in (no error)"=w499, "Message Data"=w494, "Message"="Test Tree Save State", "Message Queue"=w493) -> ("error out"=w498:errorcluster[], "dup Message Queue"=w492:refnum<queue>)  [unwired: 6 in]
            n231 = call-poly "Enqueue Message.vi"("error in (no error)"=w498, "Message"="Refresh Test Script", "Message Queue"=w492) -> ("error out"=w501:errorcluster[])  [unwired: 7 in, 1 out]
          }
        }
      }
      frame "----Messsages from Main Framework----" {
      }
      frame "Stop One Module" {
        n232 = Variant To Data(type="", Variant=w514) -> (data=w512:string)  [unwired: 1 in, 1 out]
        n233 = call "GetSetTestClass.vi"() -> ("Test.lvclass"=w511:refnum<class "Test.lvclass">)  [unwired: 11 in]
        n234 = call "StopModByName.vi"("ErrorArray In"=w515, "Module Name"=w512, "Test.lvclass"=w511) -> ("ErrorArray Out"=w506:errorcluster[], "Module Stopped"=w507:bool, "Module Name out"=w508:string, "Test.lvclass"=w510:refnum<class "Test.lvclass">)  [unwired: 5 in]
        n235 = call "GetSetTestClass.vi"("Set"=TRUE, "Test.lvclass"=w510) -> ("Test.lvclass"=w504:refnum<class "Test.lvclass">)  [unwired: 9 in]
        n236 = case shown="True" w507 {
          tunnel: w508 -> [_ w533]
          tunnel: w506 -> [w516 w532]
          tunnel: [w516 w527] -> w505
          tunnel: w504 -> [_ w519]
          frame False {
          }
          frame True {
            n237 = property class="Test.lvclass"(reference=w519) -> ("Accessors:ModuleList"=w518:string[])  [unwired: 1 in, 2 out]
            n238 = call "cntlRefs.vi"() -> ("cntlRefs"=w525:T4)  [unwired: 10 in, 1 out]
            n239 = Unbundle By Name(w525) -> ("cmbxRunningModules"=w524:refnum<vi>, "btnPopInOut"=w523:refnum<vi>)
            n240 = call "VisualizationManager.vi"("Action"=VisualizationManagerActions."CloseVisMod", "Module Name"=w533) -> ("error out"=w531:errorcluster, "In SubPanel?"=w522:bool, "Module Name out"=w521:string)  [unwired: 6 in, 1 out]
            n241 = call <userlib>:"AddError.vi"("Severity"="Warning", "Priority"=u8 2, "ErrorArray In"=w532, "error in (no error)"=w531) -> ("ErrorArray Out"=w528:errorcluster[])  [unwired: 6 in, 1 out]
            n242 = call "SetGetModuleList.vi"("Set? (F)"=TRUE, "ModuleList"=w518) -> ("ModuleList"=w520:string[])  [unwired: 9 in]
            n243 = Empty Array?(array=w520) -> (empty?=w526:bool)
            n244 = case shown="False" w526 {
              tunnel: w528 -> [_ w546]
              tunnel: [w535 w545] -> w527
              tunnel: w524 -> [w544 _]
              tunnel: w523 -> [w543 _]
              tunnel: w522 -> [w542 _]
              tunnel: w521 -> [w541 _]
              tunnel: w520 -> [w540 _]
              frame False {
                n245 = property class="Bool"(reference=w543, "Value"=w542) -> (error out=w539:errorcluster)  [unwired: 1 in, 1 out]
                n246 = property class="CmbBox"(reference=w544, error in=w539, "Strings[]"=w540, "Value"=w541) -> (error out=w536:errorcluster)  [unwired: 1 out]
                n247 = call <userlib>:"AddError.vi"("Severity"="Warning", "Priority"=u8 2, "error in (no error)"=w536) -> ("ErrorArray Out"=w535:errorcluster[])  [unwired: 7 in, 1 out]
              }
              frame True {
                n248 = call "Enqueue.vi"("ErrorArray"=w546, "Message"="All Tests Stopped") -> ("ErrorArray"=w545:errorcluster[])  [unwired: 9 in]
              }
            }
          }
        }
      }
      frame "----Running & Stopping Tests----" {
      }
      frame "RunOneTest" {
        n249 = call "cntlRefs.vi"() -> ("cntlRefs"=w555:T4)  [unwired: 10 in, 1 out]
        n250 = Unbundle By Name(w555) -> ("btnHide"=w554:refnum<vi>)
        n251 = Variant To Data(type=string[] [] ("All Tags"), Variant=w557) -> (data=w559:string[])  [unwired: 1 in, 1 out]
        n252 = property class="Bool (strict)"(reference=w554) -> ("Value"=w553:bool)  [unwired: 1 in, 2 out]
        n253 = local read "tstFilePath"() -> (w558:path)
        n254 = call "RunOneTest.vi"("ShowPanel? (f)"=w553, ".tst file"=w558, "Error Array In"=w556, "TestTreeTags"=w559) -> ("ErrorArray Out"=w551:errorcluster[], "TDMS Log File"=w549:path)  [unwired: 6 in]
        n255 = call "Enqueue.vi"("ErrorArray"=w551, "Message Data"=w549, "Message"="Test Started") -> ("ErrorArray"=w550:errorcluster[])  [unwired: 8 in]
      }
      frame "Stop All Running Tests" {
        n256 = call "GetSetTestClass.vi"() -> ("Test.lvclass"=w565:refnum<class "Test.lvclass">)  [unwired: 11 in]
        n257 = call "StopMods.vi"("ErrorArray In"=w564, "Test.lvclass"=w565) -> ("ErrorArray Out"=w563:errorcluster[])  [unwired: 8 in, 1 out]
        n258 = call "Enqueue.vi"("ErrorArray"=w563, "Message"="All Tests Stopped") -> ("ErrorArray"=w562:errorcluster[])  [unwired: 9 in]
      }
      frame "Transmit Test Run Confirmation" {
        w566 = errorcluster {"status"=FALSE, "code"=0, "source"=""} ("error constant")
        n259 = case shown="False" "Create Error (Test Python Multirun)" {
          tunnel: [_ "Error In"] -> _
          frame False {
          }
          frame True {
            (unwired) errorcluster {"status"=FALSE, "code"=0, "source"=""} ("Error In")
          }
        }
        n260 = Flatten To XML(anything=w566) -> (xml string=w572:string)
        n261 = local read "Severity"() -> (w567:string)
        n262 = call "Transmitter.vi"("ErrorArray"=w568, "XMLData"=w572, "Command"="LtaRunComplete") -> ("ErrorArray"=w571:errorcluster[])  [unwired: 7 in, 1 out]
        n263 = call <userlib>:"AddError.vi"("Severity"=w567, "Priority"=u8 2, "ErrorArray In"=w571, "error in (no error)"=w566) -> ("ErrorArray Out"=w569:errorcluster[])  [unwired: 6 in, 1 out]
      }
      frame "----Cosmetics----" {
      }
      frame "Resize Test Listbox Column" {
        n264 = call "cntlRefs.vi"() -> ("cntlRefs"=w582:T4)  [unwired: 10 in, 1 out]
        n265 = Unbundle By Name(w582) -> ("TestListboxRef"=w581:refnum<vi>)
        n266 = property on="TestListboxPane" class="Pane"() -> ("Width"=w579:u32)  [unwired: 2 in, 2 out]
        n267 = Multiply(x=w579, y=1.25) -> (x*y=w577:dbl)
        n268 = property class="MCListbox"(reference=w581, "ActiveCell"=T8 {"Row"=0, "Column"=0} ("Active Cell:Active Cell"), "Width"=w577) -> ()  [unwired: 1 in, 2 out]
      }
    }
    n269 = call "Handle Error.vi"("ErrorArrayIn"=w215, "Message Queue"=w207) -> ("ErrorArrayOut"=w214:errorcluster[])  [unwired: 9 in]
  }
  n270 = Unregister For Events(event registration refnum=w2) -> (error out=w1:errorcluster)  [unwired: 1 in]
  n271 = call <userlib>:"AddError.vi"("Severity"="Fatal", "Priority"=u8 0, "ErrorArray In"=w18, "error in (no error)"=w1) -> ("ErrorArray Out"=w17:errorcluster[])  [unwired: 6 in, 1 out]
  n272 = Merge Errors(w17, w21, w10) -> (→"Error Out":errorcluster)
